vi "generate-fault.vi"(10 "Enum in":T1, 11 "Numeric":i32) -> (3 "Enum out":T1)   [LabVIEW 2017, in "Library.lvlib"]
uses:
  Library.lvlib
  state.ctl
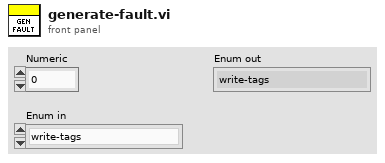
[diagram p1: front panel]
types:
  T1 = typedef "Library.lvlib/state.ctl" = enum16{"write-tags", "clear-fault", "generate-fault", "handle-error"}
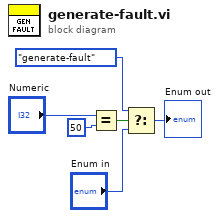
[diagram p0: block diagram]
diagram:
  n1 = Equal?(x="Numeric", y=50) -> (x = y?=w3:bool)
  n2 = Select(t=state."generate-fault", s=w3, f="Enum in") -> (s? t:f=→"Enum out":T1)
